vi "get_data.vi"(7 "LabVIEW Web Service Request":refnum<class "Web Request.lvclass">) -> ()   [LabVIEW 2014]
uses:
  <vilib>/wsapi/Web Request.lvclass
  DataManager/StateStore/Controls/DataFunction.ctl
panel:
  out "error out":errorcluster
  # "Use the Web Service Request input terminal to call the VIs on the Web Services palette. Do not remove it from the connector pane unless you don't need access to the palette."
  # "Each additional control wired to the connector pane will be available as an input in the URL. To include an indicator in terminal-mode output (the default setting), it must also be wired to the connector pane."
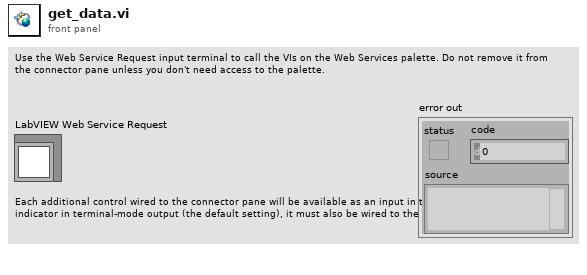
[diagram p1: front panel]
types:
  T1 = typedef "DataFunction.ctl" = enum16{"Initialise", "Release", "Get Data", "Set Data", "Preview Data"}
  T2 = typedef "CData Core Control.ctl" = cluster{"train_data_array":cluster{"uuid":string, "int":i32, "posit_array":cluster{"x":dbl, "y":dbl, "z":dbl}[]}[], "train_control_array":cluster{"uuid":string, "throttle":dbl, "brake":dbl, "horn":dbl, "wait":dbl, "name":string, "mode":string, "dest":string}[], "switch_data_array":cluster{"switch_posit":cluster{"x":dbl, "y":dbl, "z":dbl}, "manual":bool}[], "switch_control_array":cluster{"switch_posit":cluster{"x":dbl, "y":dbl, "z":dbl}, "switch":bool, "invert":bool, "wait":dbl}[]}
  T3 = cluster{"uuid":string, "int":i32, "posit_array":cluster{"x":dbl, "y":dbl, "z":dbl}[]}[]
  T4 = cluster{"switch_posit":cluster{"x":dbl, "y":dbl, "z":dbl}, "manual":bool}[]
  T5 = cluster{"train_data_array":cluster{"uuid":string, "int":i32, "posit_array":cluster{"x":dbl, "y":dbl, "z":dbl}[]}[], "switch_data_array":cluster{"switch_posit":cluster{"x":dbl, "y":dbl, "z":dbl}, "manual":bool}[]}
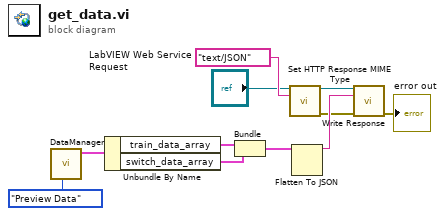
[diagram p0: block diagram]
diagram:
  n1 = call "DataManager.vi"("DataFunction"=DataFunction."Preview Data") -> ("CData Out"=w10:T2)  [unwired: 9 in, 1 out]
  n2 = Unbundle By Name(w10) -> ("train_data_array"=w8:T3, "switch_data_array"=w7:T4)
  n3 = Bundle("train_data_array"=w8, "switch_data_array"=w7) -> (w6:T5)  [unwired: 1 in]
  n4 = call <vilib>:"Set HTTP Response MIME Type.vi"("LabVIEW Web Service Request"="LabVIEW Web Service Request", "MIME type (text/html)"="text/JSON") -> ("LabVIEW Web Service Request out"=w3:refnum<class "Web Request.lvclass">, "error out"=w2:errorcluster)  [unwired: 12 in]
  n5 = Flatten To JSON(anything=w6) -> (JSON string=w9:string)  [unwired: 2 in, 1 out]
  n6 = call <vilib>:"Write Response.vi"("LabVIEW Web Service Request"=w3, "response string"=w9, "error in (no error)"=w2) -> ("error out"=→"error out":errorcluster)  [unwired: 11 in, 1 out]
